vi "Read_async_slaves_PN.vi"(5 "slaves tasks":i32[](array[numeric]), 7 "slaves buffer sizes":i32[](array[numeric]), 9 "slave N channels":u32[](array[numeric]), 11 "Samples Per Channel":i32=-1, 12 "Timeout":dbl=10.0) -> (6 "slaves tasks out":i32[](array[numeric]), 10 "slaves data":dbl[][][](array[numeric]), 15 "error out":errorcluster)   [LabVIEW 2011]
uses:
  <userlib>/LV-Link3/PolySubVIs/DtOLReadMultiple2D.vi
  <userlib>/LV-Link3/PolySubVIs/DtOLStartNormal.vi
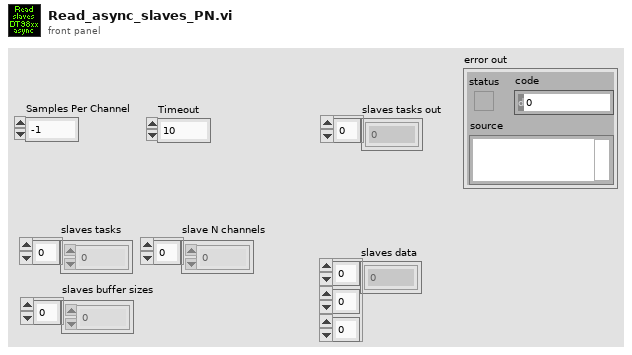
[diagram p1: front panel]
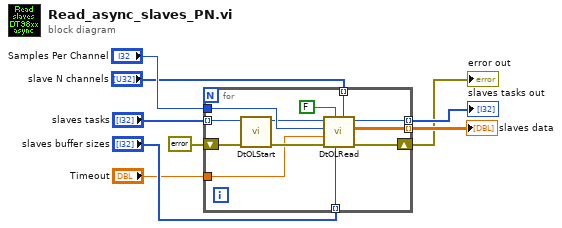
[diagram p0: block diagram]
diagram:
  n1 = for {
    tunnel: [w21] -> w5 mode=indexing
    tunnel: [w17] -> w4 mode=indexing
    shift-right: [w16] -> w2
    shift-left: errorcluster {"status"=FALSE, "code"=0, "source"=""} ("error in (no error)") -> [w15]
    tunnel: "slaves tasks" -> [w11] mode=indexing
    tunnel: "slaves buffer sizes" -> [w19] mode=indexing
    tunnel: "Samples Per Channel" -> [w13]
    tunnel: "slave N channels" -> [w18] mode=indexing
    tunnel: "Timeout" -> [w10]
    n2 = call-poly <userlib>:"DtOLStart.vi"("error in (no error)"=w15, "Task in"=w11) -> ("error out"=w14:errorcluster, "Task out"=w12:i32)  [unwired: 8 in]
    n3 = call-poly <userlib>:"DtOLRead.vi"("Number Chan to Read"=w18, "Buffer size"=w19, "OnlyReadAvailable"=FALSE, "error in (no error)"=w14, "Timeout"=w10, "Samples Per Channel"=w13, "Task in"=w12) -> ("error out"=w16:errorcluster, "2D Data out"=w21:dbl[][], "Task out"=w17:i32)  [unwired: 2 out]
  }
  "error out" <- w2
  "slaves data" <- w5
  "slaves tasks out" <- w4
